vi "AccelnetVelInScale.vi"(1 "Acelnet eCAT vel":i32) -> (0 "Shaft vel (rad/s)":dbl)   [LabVIEW 2018]
uses:
  Clusters/SimulationConstants.ctl
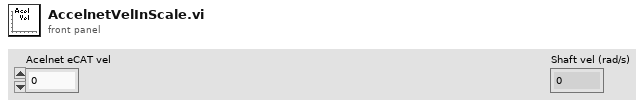
[diagram p1: front panel]
types:
  T1 = typedef "SimulationConstants.ctl" = cluster{"nGear":dbl, "rotorRadius":sgl, "numBlades":i32, "scaleFactor":dbl, "roscoInitMinSpeed_rad_s":dbl, "roscoInitMinTorqueFS_Nm":dbl, "beckhoff24BitExt":i32, "torqueCellFullV":dbl, "torqueCellFullNm":dbl, "torqueCellELM3148V":dbl, "nacelleAccELM3604V":dbl, "nacelleAccScaleX":dbl, "nacelleAccOfstX":dbl, "nacelleAccScaleY":dbl, "nacelleAccOfstY":dbl, "nacelleAccScaleZ":dbl, "nacelleAccOfstZ":dbl, "cyberGearRatio":dbl, "cyberLinesPerRev":dbl, "cyberRatedTorque":dbl}
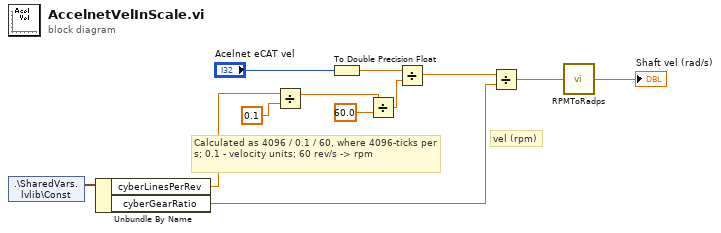
[diagram p0: block diagram]
diagram:
  # "vel (rpm)"
  # "Calculated as 4096 / 0.1 / 60, where 4096-ticks per s; 0.1 - velocity units; 60 rev/s -> rpm"
  n1 = shared-variable ".\\SharedVars.lvlib\\Const"() -> (w7:T1)  [unwired: 1 in, 1 out]
  n2 = Unbundle By Name(w7) -> ("cyberLinesPerRev"=w5:dbl, "cyberGearRatio"=w6:dbl)
  n3 = Divide(x=w5, y=0.1) -> (x/y=w3:dbl)
  n4 = To Double Precision Float(number="Acelnet eCAT vel") -> (double precision float=w12:dbl)
  n5 = Divide(x=w3, y=60.0) -> (x/y=w1:dbl)
  n6 = Divide(x=w12, y=w1) -> (x/y=w11:dbl)
  n7 = Divide(x=w11, y=w6) -> (x/y=w9:dbl)
  n8 = call "RPMToRadps.vi"("rpm"=w9) -> ("rad/s"=→"Shaft vel (rad/s)":dbl)
